vi "Test All.vi"(11 "Error in":errorcluster) -> (15 "Error out":errorcluster)   [LabVIEW 2020, in "CelsiusToFarenheitTests.lvlib"]
doc: "This vi runs all the test cases for the Celsius to Fahrenheit assignment. Also the test report gets saved as a xml format.\n\n* USES *\nDrona, G-CLI and Caraya"
uses:
  CelsiusToFarenheitTests.lvlib
  <vilib>/addons/_JKI Toolkits/Caraya/classes/Test Suite/Define Test Suite (JUnit Report).vi
  <vilib>/Utility/error.llb/Error Cluster From Error Code.vi
  <vilib>/ErrorRing/Error Ring.xnode
  <vilib>/addons/_JKI Toolkits/Caraya/classes/Test Suite/Test Suite.lvclass
  <vilib>/addons/_JKI Toolkits/Caraya/classes/Test/Test.lvclass
  <vilib>/Wiresmith Technology/G CLI/CLI Class/CLI.lvclass
  <vilib>/addons/_JKI Toolkits/Caraya/classes/Test Result/Test Result.lvclass
panel:
  # "TESTING ALL TEST CASES FOR CELSIUS TO FAHRENHEIT"
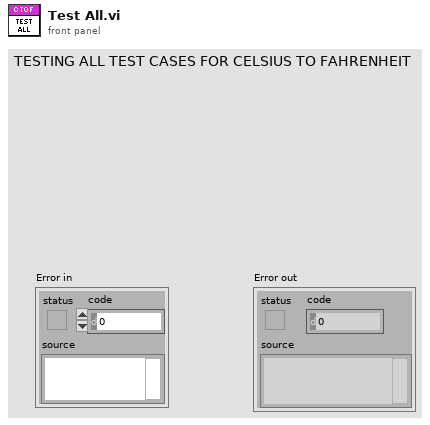
[diagram p1: front panel]
types:
  T1 = typedef "Caraya.lvlib/Test Result.lvclass/Node Results.ctl" = cluster{"Node":T2, "Assertions":T4[]}
  T2 = typedef "Caraya.lvlib/Test Result.lvclass/Test Node.ctl" = cluster{"Test Registration":T3, "Defined":bool, "Passed":bool}
  T3 = typedef "Caraya.lvlib/Test Result.lvclass/Test Registration Data.ctl" = cluster{"Name":string, "Call Chain":string[], "Time Stamp":timestamp, "Test ID":string, "Caller ID":string}
  T4 = typedef "Caraya.lvlib/Test Result.lvclass/Assert Event Data.ctl" = cluster{"Name":string, "Passed":bool, "Call Chain":string[], "Test Error":errorcluster, "Time Stamp":timestamp, "Unique Assert ID":string, "Test ID":string, "Execution time (s)":dbl, "Verbose Explanation":string}
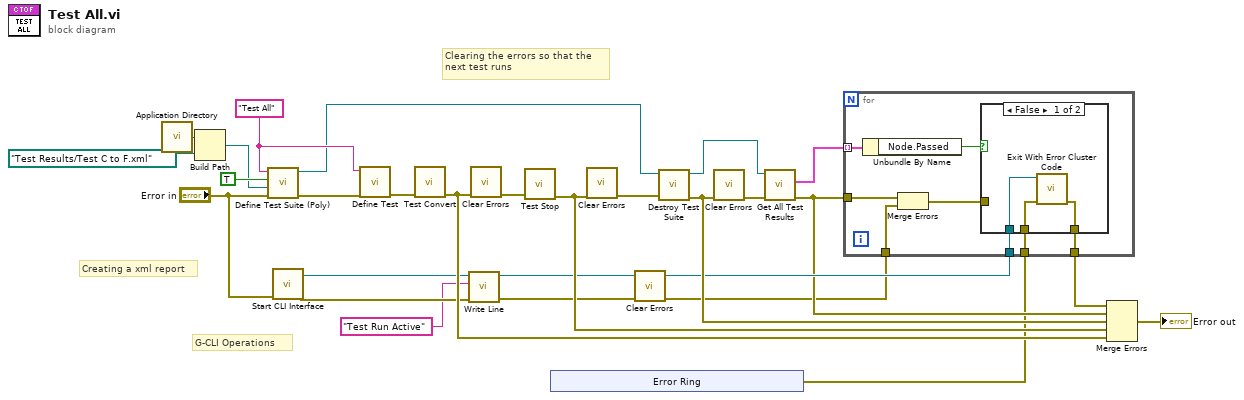
[diagram p0: block diagram]
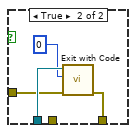
[diagram p2: hidden frame]
diagram:
  w22 = "Test All" ("Label (VI Title)")
  # "G-CLI Operations"
  # "Creating a xml report"
  # "Clearing the errors so that the\nnext test runs"
  n1 = call <vilib>:"Application Directory.vi"() -> ("Application Directory"=w27:path)
  n2 = Build Path(base path=w27, name or relative path=path "Test Results/Test C to F.xml") -> (appended path=w24:path)
  n3 = call-poly <vilib>:"Define Test Suite (Poly).vi"("error in (no error)"="Error in", "Report Path"=w24, "Interactive"=TRUE, "Label (VI Title)"=w22) -> ("error out"=w23:errorcluster, "Test Suite"=w21:refnum<class "Test Suite.lvclass">)  [unwired: 6 in]
  n4 = call <vilib>:"Start CLI Interface.vi"("error in (no error)"="Error in") -> ("error out"=w13:errorcluster, "CLI out"=w11:refnum<class "CLI.lvclass">)  [unwired: 7 in, 2 out]
  n5 = call <vilib>:"Define Test.vi"("error in (no error)"=w23, "Label (VI Title)"=w22) -> ("error out"=w20:errorcluster)  [unwired: 9 in]
  n6 = call "Test Convert.vi"("Error in"=w20) -> ("Error out"=w17:errorcluster)  [unwired: 14 in]
  n7 = call <vilib>:"Write Line.vi"("error in (no error)"=w13, "Text to Write"="Test Run Active", "CLI in"=w11) -> ("error out"=w3:errorcluster, "CLI out"=w6:refnum<class "CLI.lvclass">)  [unwired: 7 in]
  n8 = call <vilib>:"Clear Errors.vi"("error in (no error)"=w17) -> ("error out"=w19:errorcluster)  [unwired: 5 in, 1 out]
  n9 = call "Test Stop.vi"("Error in"=w19) -> ("Error out"=w16:errorcluster)  [unwired: 14 in]
  n10 = xnode "Error Ring"() -> ("error out"=w1:errorcluster)
  n11 = call <vilib>:"Clear Errors.vi"("error in (no error)"=w16) -> ("error out"=w18:errorcluster)  [unwired: 5 in, 1 out]
  n12 = call <vilib>:"Clear Errors.vi"("error in (no error)"=w3) -> ("error out"=w2:errorcluster)  [unwired: 5 in, 1 out]
  n13 = call-dynamic "Destroy Test Suite.vi"("error in (no error)"=w18, "Test Suite in"=w21) -> ("error out"=w7:errorcluster, "Test Suite Results"=w9:refnum<class "Test Result.lvclass">)  [unwired: 8 in]
  n14 = call <vilib>:"Clear Errors.vi"("error in (no error)"=w7) -> ("error out"=w8:errorcluster)  [unwired: 5 in, 1 out]
  n15 = call <vilib>:"Get All Test Results.vi"("error in (no error)"=w8, "Test Result in"=w9) -> ("error out"=w4:errorcluster, "Test Results"=w10:T1[])  [unwired: 7 in, 1 out]
  n16 = for {
    tunnel: w10 -> [w35] mode=indexing
    tunnel: w6 -> [w33]
    tunnel: [w32] -> w5
    tunnel: w4 -> [w31]
    tunnel: w2 -> [w30]
    tunnel: w1 -> [w28]
    n17 = Unbundle By Name(w35) -> ("Node.Passed"=w34:bool)
    n18 = Merge Errors(w31, w30) -> (w29:errorcluster)
    n19 = case shown="False" w34 {
      tunnel: w33 -> [w38 w42]
      tunnel: [w37 w40] -> w32
      tunnel: w29 -> [_ w39]
      tunnel: w28 -> [w36 _]
      frame False {
        n20 = call <vilib>:"Exit With Error Cluster Code.vi"("error in (no error)"=w36, "CLI in"=w38) -> ("error out"=w37:errorcluster)  [unwired: 9 in]
      }
      frame True {
        n21 = call <vilib>:"Exit with Code.vi"("error in (no error)"=w39, "Exit Code (0)"=0, "CLI in"=w42) -> ("error out"=w40:errorcluster)  [unwired: 8 in]
      }
    }
  }
  n22 = Merge Errors(w5, w4, w7, w16, w17) -> (→"Error out":errorcluster)
